vi "Log Event.vi"(8 "error in (no error)":errorcluster, 10 "Debug Data.lvclass":refnum<class "Debug Data.lvclass">, 11 "Debugger In":refnum<class "Debugger.lvclass">) -> (0 "error out":errorcluster, 2 "Debug Data out":refnum<class "Debug Data.lvclass">, 3 "Debugger Out":refnum<class "Debugger.lvclass">)   [LabVIEW 2020, in "Debugger.lvclass"]
uses:
  Debugger.lvclass
  Debug Data/Debug Data.lvclass
  Debugger.lvclass/Debugger.ctl
  Debug Log/Debug Log.lvclass
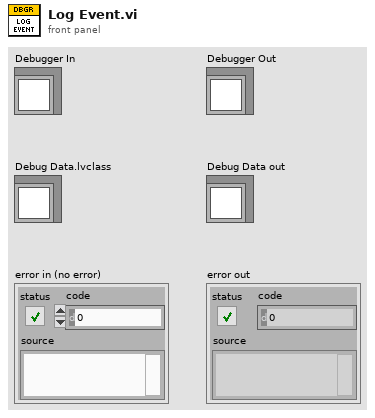
[diagram p1: front panel]
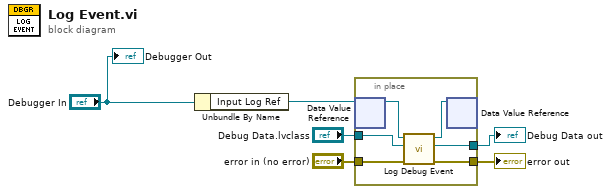
[diagram p0: block diagram]
diagram:
  n1 = Unbundle By Name("Debugger In") -> ("Input Log Ref"=w1:refnum<data-value>)
  n2 = in-place {
    in-place-border: [w12] -> w5
    in-place-border: "Debug Data.lvclass" -> [w11]
    in-place-border: [w10] -> w3
    in-place-border: "error in (no error)" -> [w9]
    n3 = in-place-dvr #1(w1) -> (w8:refnum<class "Debug Log.lvclass">)  [unwired: 1 out]
    n4 = call "Log Debug Event.vi"("error in (no error)"=w9, "Debug Data.lvclass"=w11, "Debugger in"=w8) -> ("error out"=w10:errorcluster, "Debug Data Out"=w12:refnum<class "Debug Data.lvclass">, "Debugger out"=w7:refnum<class "Debug Log.lvclass">)  [unwired: 6 in]
    n5 = in-place-dvr #1(w7) -> ()  [unwired: 2 out]
  }
  "Debug Data out" <- w5
  "error out" <- w3
  "Debugger Out" <- "Debugger In"
